vi "QueryComandList.vi"(8 "Fehler (Eingang, kein Fehler)":errorcluster caption="Error_In", 11 "OXYGEN Ref In":refnum<visa-resource-name>) -> (0 "Fehler (Ausgang)":errorcluster caption="Error_Out", 1 "communication_data":T1, 2 "commands as list":string[](array[string]), 3 "OXYGEN Ref Out":refnum<visa-resource-name>, 4 "num char":i32)   [LabVIEW 2018, in "OXYGEN.lvlib"]
doc: "Queries the implemented commands as list"
uses:
  OXYGEN.lvlib
  TypeDefs/Cluster_RawCommData.ctl
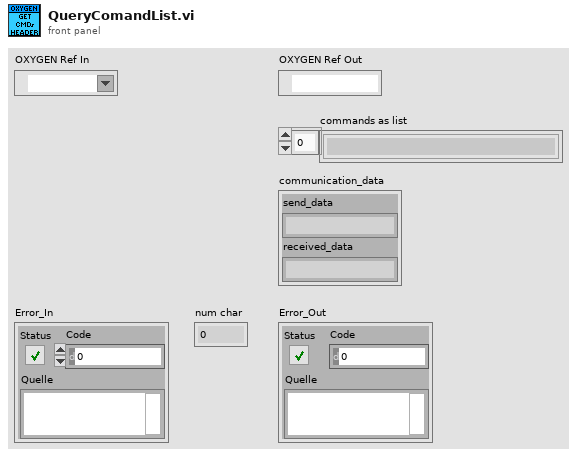
[diagram p1: front panel]
types:
  T1 = typedef "OXYGEN.lvlib/Cluster_RawCommData.ctl" = cluster{"send_data":string, "received_data":string}
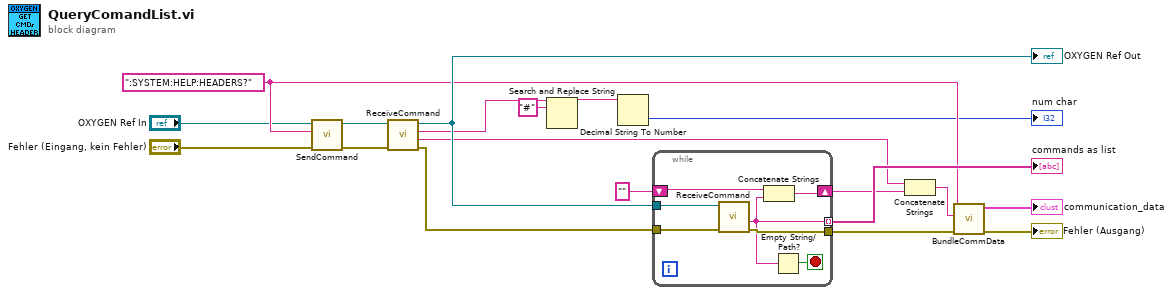
[diagram p0: block diagram]
diagram:
  w4 = ":SYSTEM:HELP:HEADERS?" ("Schreibpuffer")
  n1 = call "SendCommand.vi"("error in (no error)"="Fehler (Eingang, kein Fehler)", "String to Send"=w4, "OXY_SCPI Reseource In"="OXYGEN Ref In") -> ("error out"=w19:errorcluster, "OXY_SCPI Reseource Out"=w18:refnum<visa-resource-name>)  [unwired: 7 in]
  n2 = call "ReceiveCommand.vi"("error in (no error)"=w19, "OXY_SCPI Reseource In"=w18) -> ("error out"=w11:errorcluster, "received Data with Header"=w5:string, "received Data"=w8:string, "OXY_SCPI Reseource Out"=w13:refnum<visa-resource-name>)  [unwired: 6 in]
  "OXYGEN Ref Out" <- w13
  n3 = Search and Replace String(input string=w8, search string="#") -> (result string=w14:string)  [unwired: 6 in, 3 out]
  n4 = Decimal String To Number(string=w14) -> (number=→"num char":i32)  [unwired: 2 in, 1 out]
  n5 = while {
    tunnel: w13 -> [w26]
    tunnel: [w21] -> w12 mode=indexing
    tunnel: w11 -> [w24]
    tunnel: [w23] -> w10
    shift-right: [w20] -> w7
    shift-left: "" -> [w22]
    stop <- w25 stop-if-true
    n6 = call "ReceiveCommand.vi"("error in (no error)"=w24, "OXY_SCPI Reseource In"=w26) -> ("error out"=w23:errorcluster, "received Data with Header"=w21:string)  [unwired: 6 in, 2 out]
    n7 = Concatenate Strings(w22, w21) -> (w20:string)
    n8 = Empty String/Path?(string/path=w21) -> (empty?=w25:bool)
  }
  "commands as list" <- w12
  n9 = Concatenate Strings(w5, w7) -> (w6:string)
  n10 = call "BundleCommData.vi"("error in (no error)"=w10, "received_data"=w6, "send_data"=w4) -> ("error out"=→"Fehler (Ausgang)":errorcluster, "communication_data"=→"communication_data":T1)  [unwired: 7 in]
